vi "Min_of_3.vi"(8 "error in":errorcluster, 9 "input 02":dbl, 10 "input 01":dbl, 11 "input 03":dbl) -> (0 "error out":errorcluster, 2 "min":dbl)   [LabVIEW 2022 SP3]
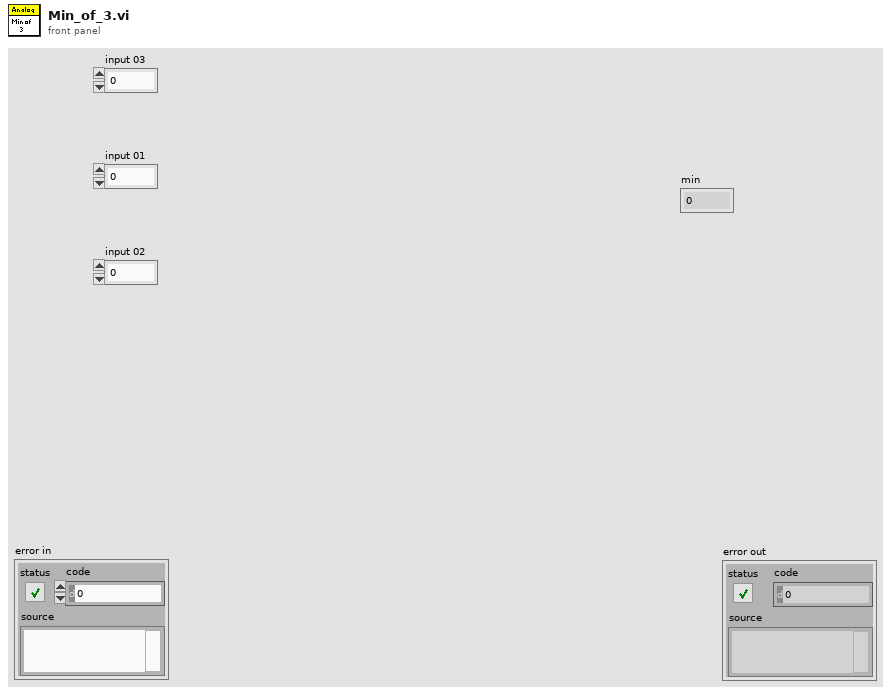
[diagram p1: front panel]
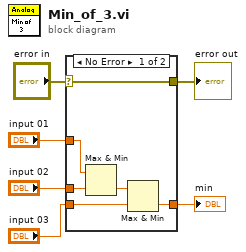
[diagram p0: block diagram]
diagram:
  n1 = case shown="No Error" "error in" {
    selector: "error in" -> [w11 w13]
    tunnel: [w11 w13] -> w5
    tunnel: "input 01" -> [w10 _]
    tunnel: "input 02" -> [w9 _]
    tunnel: "input 03" -> [w8 _]
    tunnel: [w7 _] -> w1
    frame No Error {
      n2 = Max & Min(x=w10, y=w9) -> (min(x,y)=w12:dbl)  [unwired: 1 out]
      n3 = Max & Min(x=w12, y=w8) -> (min(x,y)=w7:dbl)  [unwired: 1 out]
    }
    frame Error {
    }
  }
  "error out" <- w5
  "min" <- w1
